vi "UDP Communication.vi"(8 "error in":errorcluster) -> ()   [LabVIEW 2011]
doc: "This VI runs in parallel to other tasks. It can contain as many user-defined periodic loops as you need. These can carry out PID or other sorts of timed response."
uses:
  UDP Dashboard Packet TypeDef.ctl
  Robot Global Data.vi
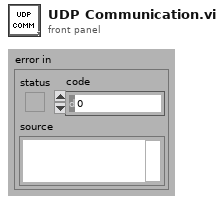
[diagram p1: front panel]
types:
  T1 = typedef "UDP Dashboard Packet TypeDef.ctl" = cluster{"Distance":dbl, "Shooter Control":cluster{"Manual Enabled":bool, "Manual Distance":dbl, "Power Constant":dbl, "RPM Constant":dbl, "Layup Distance":dbl, "RPM Range":cluster{"Max Percentage":dbl, "Min Percentage":dbl}, "Dt In":dbl}, "Tracking Setpoint":dbl, "Shooter PID gains":cluster{"proportional gain (Kc)":dbl, "integral time (Ti, min)":dbl, "derivative time (Td, min)":dbl}, "Tracking PID gains":cluster{"proportional gain (Kc)":dbl, "integral time (Ti, min)":dbl, "derivative time (Td, min)":dbl}, "Shooter PID gains 2":cluster{"proportional gain (Kc)":dbl, "integral time (Ti, min)":dbl, "derivative time (Td, min)":dbl}, "Tracking Tolerance":dbl, "Tracking Limit":dbl, "Autonomous Ball Collection / Shoot Period":dbl}
  T2 = typedef "WPI_JoystickButtonState.ctl" = cluster{"Button 1":bool, "Button 2":bool, "Button 3":bool, "Button 4":bool, "Button 5":bool, "Button 6":bool, "Button 7":bool, "Button 8":bool, "Button 9":bool, "Button 10":bool, "Button 11":bool, "Button 12":bool}
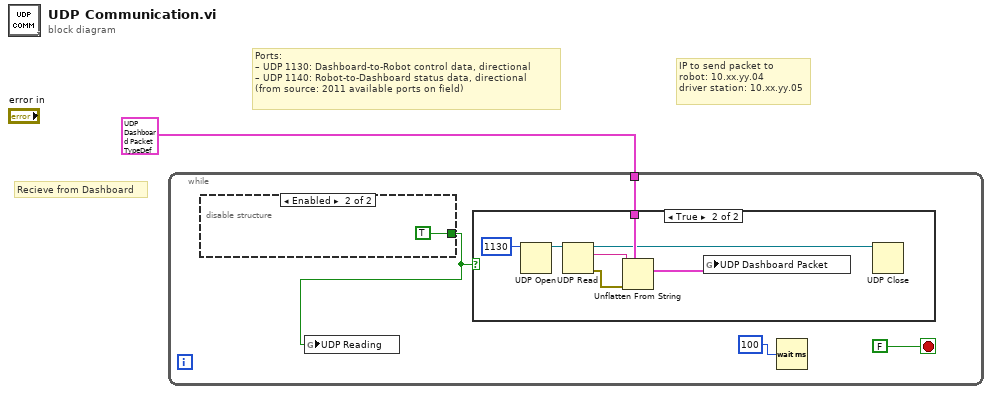
[diagram p0: block diagram]
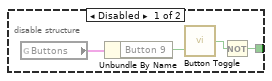
[diagram p2: hidden frame]
diagram:
  # "IP to send packet to \nrobot: 10.xx.yy.04\ndriver station: 10.xx.yy.05"
  # "Recieve from Dashboard"
  # "Ports:\n– UDP 1130: Dashboard-to-Robot control data, directional\n– UDP 1140: Robot-to-Dashboard status data, directional\n(from source: 2011 available ports on field)"
  n1 = while {
    tunnel: T1 {"Distance"=0.0, "Shooter Control"={"Manual Enabled"=FALSE, "Manual Distance"=0.0, "Power Constant"=0.0, "RPM Constant"=0.0, "Layup Distance"=0.0, "RPM Range"={"Max Percentage"=0.0, "Min Percentage"=0.0}, "Dt In"=0.0}, "Tracking Setpoint"=0.0, "Shooter PID gains"={"proportional gain (Kc)"=0.0, "integral time (Ti, min)"=0.0, "derivative time (Td, min)"=0.0}, "Tracking PID gains"={"proportional gain (Kc)"=0.0, "integral time (Ti, min)"=0.0, "derivative time (Td, min)"=0.0}, "Shooter PID gains 2"={"proportional gain (Kc)"=0.0, "integral time (Ti, min)"=0.0, "derivative time (Td, min)"=0.0}, "Tracking Tolerance"=0.0, "Tracking Limit"=0.0, "Autonomous Ball Collection / Shoot Period"=0.0} ("UDP Dashboard Packet") -> [w4]
    stop <- FALSE stop-if-true
    n2 = disable-structure shown="Enabled" {
      disable-tunnel: [w6 TRUE ("UDP Reading")] -> w2
      frame Disabled {
        n3 = global read "Robot Global Data.vi" "Buttons"() -> (w9:T2)
        n4 = Unbundle By Name(w9) -> ("Button 9"=w8:bool)
        n5 = call "Button Toggle.vi"("Button Input"=w8) -> ("Toggled Output"=w7:bool)
        n6 = Not(x=w7) -> (.not. x?=w6:bool)
      }
      frame Enabled {
      }
    }
    n7 = global write "Robot Global Data.vi" "UDP Reading"(w2) -> ()
    n8 = case shown="True" w2 {
      tunnel: w4 -> [_ w15]
      frame False {
      }
      frame True {
        n9 = UDP Open(11:u16 1130 ("port")) -> (port=w12:refnum<k16>)  [unwired: 4 in, 2 out]
        n10 = UDP Read(connection ID=w12) -> (data out=w16:string, error out=w17:errorcluster, 3:w11:refnum<k16>)  [unwired: 3 in, 2 out]
        n11 = Unflatten From String(type=w15, binary string=w16, error in (no error)=w17) -> (value=w14:T1)  [unwired: 2 in, 2 out]
        n12 = global write "Robot Global Data.vi" "UDP Dashboard Packet"(w14) -> ()
        n13 = UDP Close(connection ID=w11) -> ()  [unwired: 1 in, 2 out]
      }
    }
    n14 = Wait (ms)(milliseconds to wait=u32 100) -> ()  [unwired: 1 out]
  }
